vi "HC.vi"() -> ()   [LabVIEW 2022 SP3]
uses:
  <vilib>/numeric/Random Number (Range) I64.vi
  <vilib>/numeric/sub_Random U32.vi
panel:
  in  "TOSS":bool
  in  "Exit":bool
  in  "BOWL":bool
  in  "BAT":bool
  out "RESULT":string
  out "RUNS TO WIN":dbl
  in  "6":bool
  in  "5":bool
  in  "4":bool
  in  "3":bool
  in  "2":bool
  in  "1":bool
  out "BOT RUNS":dbl
  out "PLAYER RUNS":dbl
  out "BOWLING":dbl
  out "BATTING":dbl
  # "SCOREBOARD"
  # "SCOREBOARD"
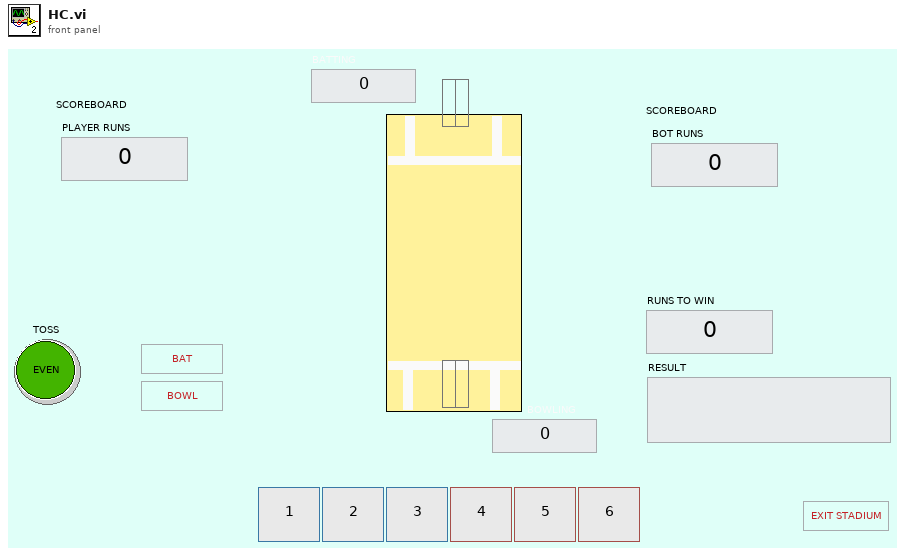
[diagram p1: front panel]
types:
  T1 = cluster{"BAT":bool, "Bowl":bool, "BATTING":dbl, "bowling":dbl, "Target":dbl, "Player Runs":dbl, "Bot Runs":dbl, "Bat CtlRef":refnum<vi>, "Choice":bool[], "RESULT":string, "Choices":dbl, "Innings switched":bool, "Random run":dbl}
  T2 = enum16{"Init", "Poll", "Bat counter", "check wicket", "result", "quit"}
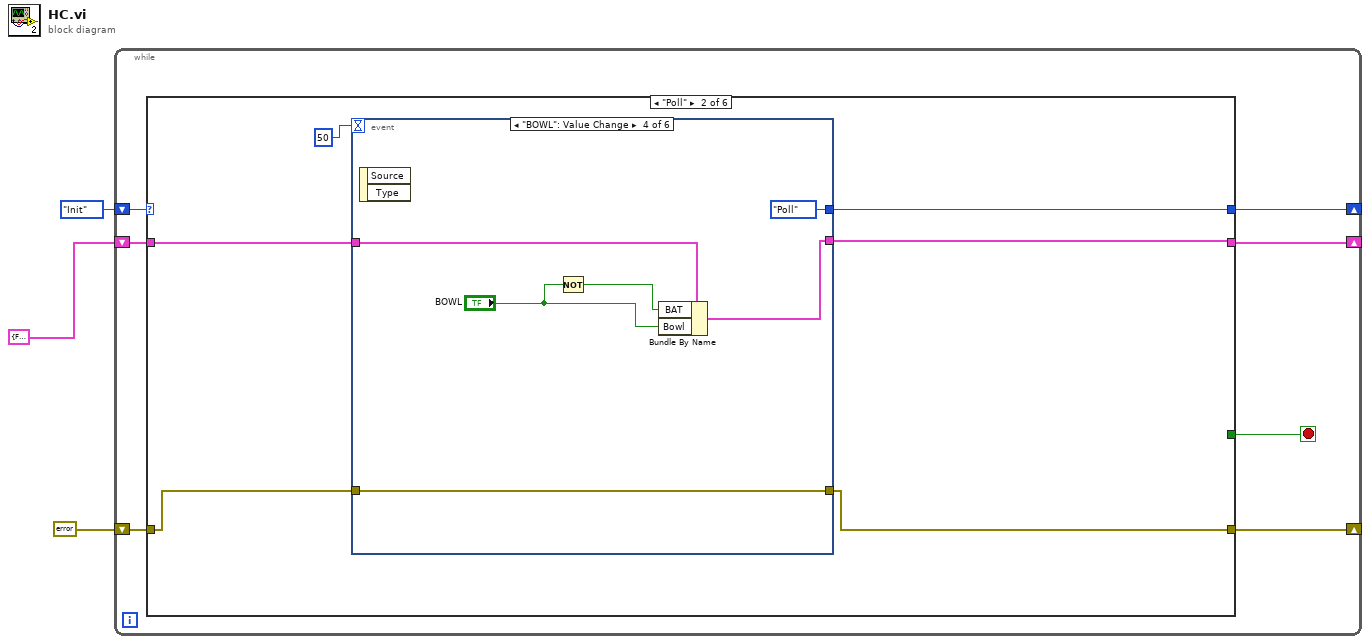
[diagram p0: block diagram]
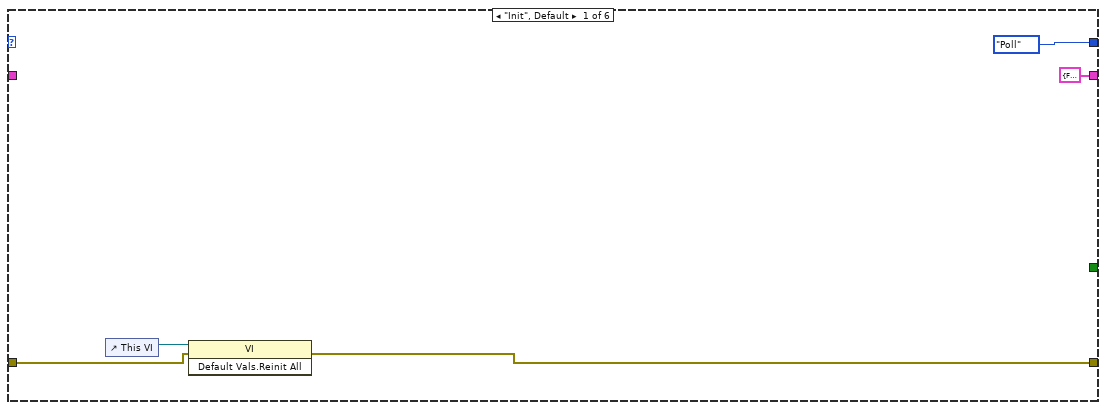
[diagram p2: hidden frame]
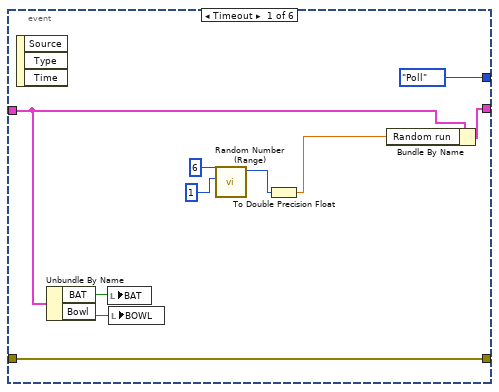
[diagram p3: hidden frame]
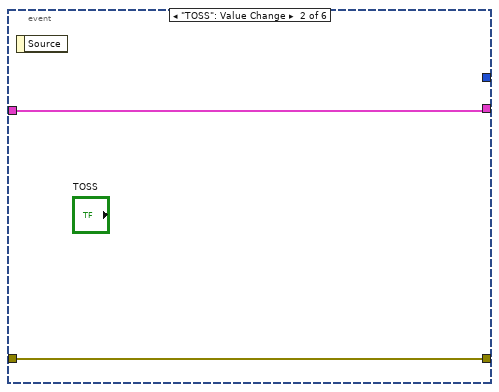
[diagram p4: hidden frame]
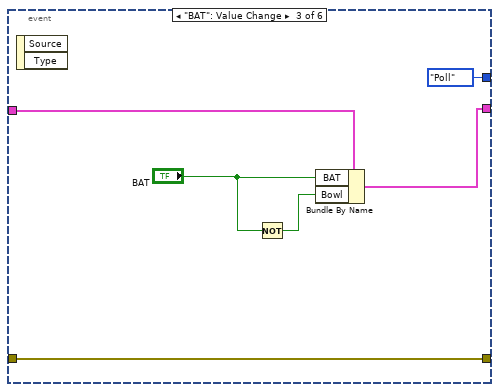
[diagram p5: hidden frame]
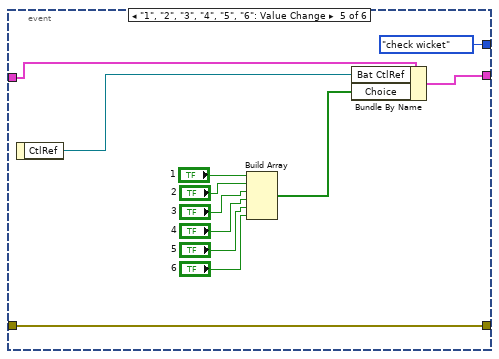
[diagram p6: hidden frame]
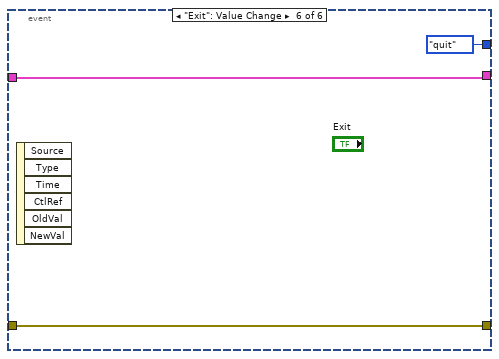
[diagram p7: hidden frame]
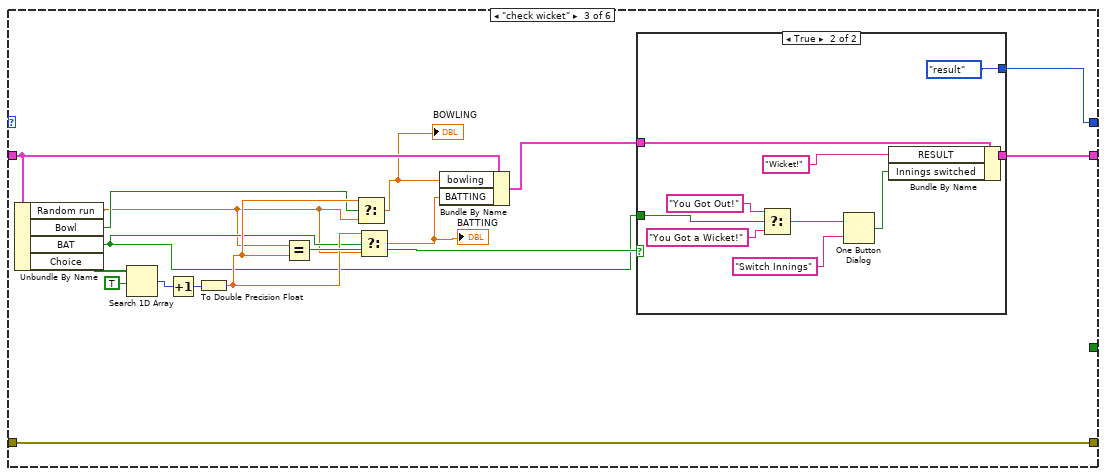
[diagram p8: hidden frame]
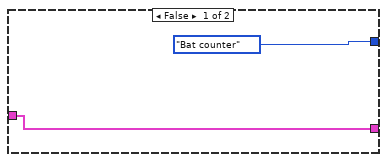
[diagram p9: hidden frame]
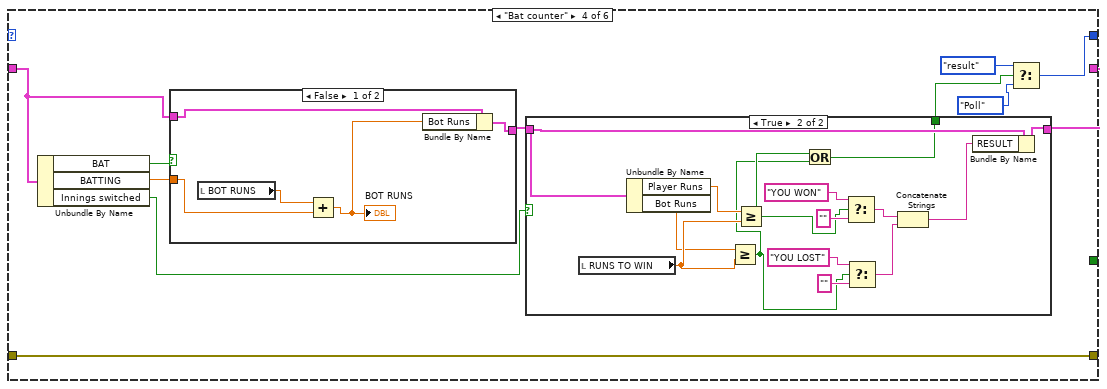
[diagram p10: hidden frame]
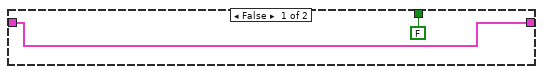
[diagram p11: hidden frame]
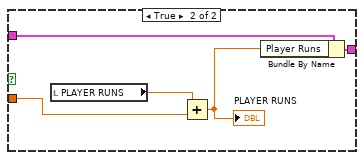
[diagram p12: hidden frame]
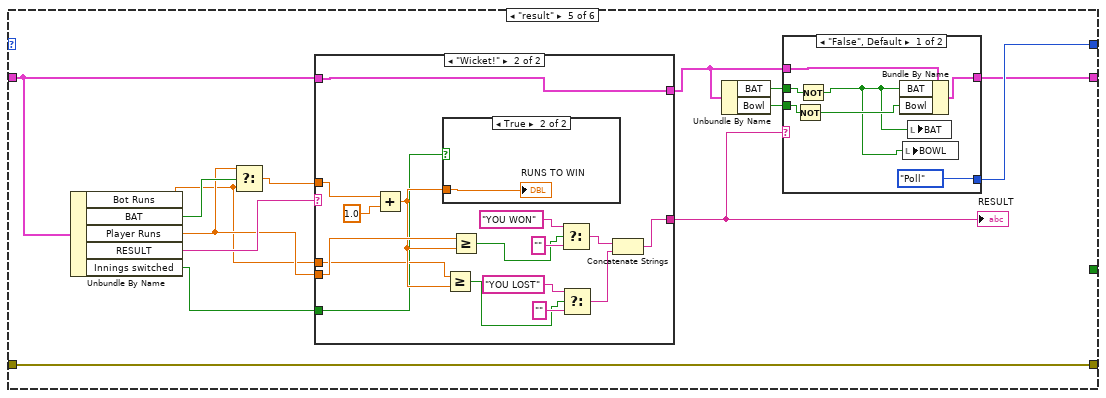
[diagram p13: hidden frame]
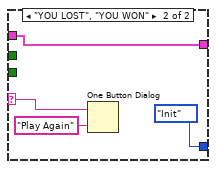
[diagram p14: hidden frame]
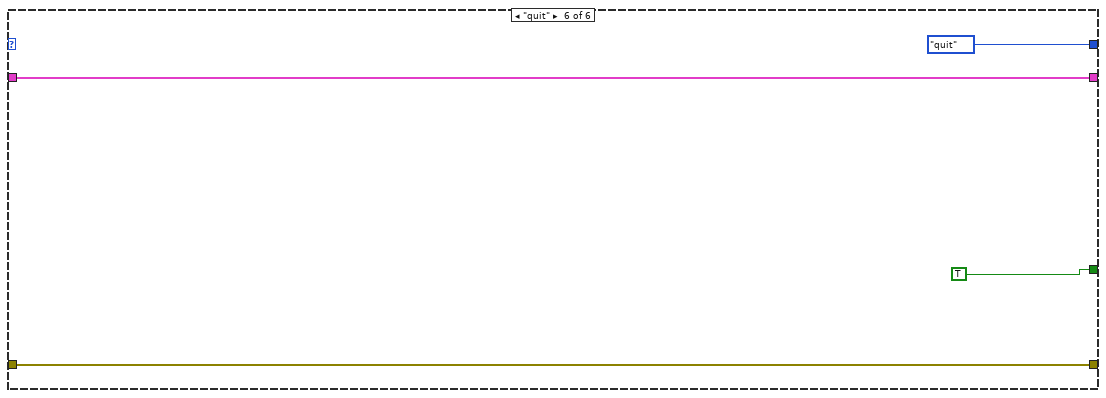
[diagram p17: hidden frame]
diagram:
  n1 = while {
    shift-right: [w9] -> _
    shift-left: T2."Init" -> [w10]
    shift-right: [w8] -> _
    shift-left: T1 {"BAT"=FALSE, "Bowl"=FALSE, "BATTING"=0.0, "bowling"=0.0, "Target"=0.0, "Player Runs"=0.0, "Bot Runs"=0.0, "Bat CtlRef"=refnum, "Choice"=[], "RESULT"="", "Choices"=0.0, "Innings switched"=FALSE, "Random run"=0.0} -> [w7]
    shift-right: [w5] -> _
    shift-left: errorcluster {"status"=FALSE, "code"=0, "source"=""} ("error in (no error)") -> [w6]
    stop <- w4 stop-if-true
    n2 = case shown="\"Poll\"" w10 {
      tunnel: [T2."Poll" ("f") w21 w72 w92 w132 T2."quit" ("f")] -> w9
      tunnel: [T1 {"BAT"=FALSE, "Bowl"=FALSE, "BATTING"=0.0, "bowling"=0.0, "Target"=0.0, "Player Runs"=0.0, "Bot Runs"=0.0, "Bat CtlRef"=refnum, "Choice"=[], "RESULT"="", "Choices"=0.0, "Innings switched"=FALSE, "Random run"=0.0} w19 w63 w94 w130 w174] -> w8
      tunnel: w7 -> [_ w20 w71 w96 w131 w174]
      tunnel: w6 -> [w14 w16 w76 w99 w140 w173]
      tunnel: [w13 w18 w76 w99 w140 w173] -> w5
      tunnel: [_ _ _ _ _ TRUE] -> w4
      frame "Init", Default {
        n3 = control-ref of="This VI"() -> (w15:refnum<vi>)
        n4 = invoke class="VI" method="Default Vals.Reinit All"(reference=w15, error in=w14) -> (error out=w13:errorcluster)  [unwired: 1 in, 2 out]
      }
      frame "Poll" {
        n5 = event shown="[3] \"BOWL\": Value Change" {
          selector: _ -> [_ _ _ _ _ _]
          dyn-events: _ -> [_ _ _ _ _ _]
          timeout: 50 -> [_ _ _ _ _ _]
          tunnel: [T2."Poll" _ T2."Poll" T2."Poll" T2."check wicket" T2."quit"] -> w21
          tunnel: [w26 w33 w37 w43 w56 w60] -> w19
          tunnel: w20 -> [w24 w33 w36 w42 w55 w60]
          tunnel: w16 -> [w30 w32 w39 w45 w53 w59]
          tunnel: [w30 w32 w39 w45 w53 w59] -> w18
          event Timeout {
            n6 = event-data() -> ()  [unwired: 1 in, 3 out]
            n7 = Unbundle By Name(w24) -> ("BAT"=w23:bool, "Bowl"=w22:bool)
            n8 = local write "BAT"(w23) -> ()
            n9 = local write "BOWL"(w22) -> ()
            n10 = call-poly <vilib>:"Random Number (Range).vi"("lower bound (-100)"=i64 1, "upper bound (100)"=i64 6) -> ("number"=w27:i64)  [unwired: 9 in]
            n11 = To Double Precision Float(number=w27) -> (double precision float=w25:dbl)
            n12 = Bundle By Name(cluster=w24, "Random run"=w25) -> (w26:T1)
          }
          event "TOSS": Value Change {
            n13 = event-data() -> ()  [unwired: 1 in, 1 out]
          }
          event "BAT": Value Change {
            n14 = event-data() -> ()  [unwired: 1 in, 2 out]
            n15 = Not(x="BAT") -> (.not. x?=w34:bool)
            n16 = Bundle By Name(cluster=w36, "BAT"="BAT", "Bowl"=w34) -> (w37:T1)
          }
          event "BOWL": Value Change {
            n17 = event-data() -> ()  [unwired: 1 in, 2 out]
            n18 = Not(x="BOWL") -> (.not. x?=w40:bool)
            n19 = Bundle By Name(cluster=w42, "BAT"=w40, "Bowl"="BOWL") -> (w43:T1)
          }
          event "1", "2", "3", "4", "5", "6": Value Change {
            n20 = event-data() -> ("CtlRef"=w54:refnum<vi>)  [unwired: 1 in]
            n21 = Build Array("1", "2", "3", "4", "5", "6") -> (w46:bool[])
            n22 = Bundle By Name(cluster=w55, "Bat CtlRef"=w54, "Choice"=w46) -> (w56:T1)
          }
          event "Exit": Value Change {
            n23 = event-data() -> ()  [unwired: 1 in, 6 out]
          }
        }
      }
      frame "check wicket" {
        n24 = Unbundle By Name(w71) -> ("Random run"=w61:dbl, "Bowl"=w67:bool, "BAT"=w62:bool, "Choice"=w75:bool[])
        n25 = Search 1D Array(1D array=w75, element=TRUE) -> (index of element=w69:i32)  [unwired: 1 in]
        n26 = Increment(x=w69) -> (x+1=w70:i32)
        n27 = To Double Precision Float(number=w70) -> (double precision float=w68:dbl)
        n28 = Equal?(x=w61, y=w68) -> (x = y?=w73:bool)
        n29 = Select(t=w68, s=w67, f=w61) -> (s? t:f=w64:dbl)
        "BOWLING" <- w64
        n30 = Select(t=w68, s=w62, f=w61) -> (s? t:f=w65:dbl)
        "BATTING" <- w65
        n31 = Bundle By Name(cluster=w71, "bowling"=w64, "BATTING"=w65) -> (w66:T1)
        n32 = case shown="True" w73 {
          tunnel: [T2."Bat counter" T2."result" ("f")] -> w72
          tunnel: [w77 w87] -> w63
          tunnel: w66 -> [w77 w86]
          tunnel: w62 -> [_ w84]
          frame False {
          }
          frame True {
            n33 = Select(t="You Got Out!" ("message"), s=w84, f="You Got a Wicket!" ("message")) -> (s? t:f=w81:string)
            n34 = One Button Dialog(message=w81, button name ("OK")="Switch Innings") -> (true=w79:bool)
            n35 = Bundle By Name(cluster=w86, "RESULT"="Wicket!", "Innings switched"=w79) -> (w87:T1)
          }
        }
      }
      frame "Bat counter" {
        n36 = Unbundle By Name(w96) -> ("BAT"=w98:bool, "BATTING"=w97:dbl, "Innings switched"=w89:bool)
        n37 = case shown="False" w98 {
          tunnel: w97 -> [w121 w125]
          tunnel: w96 -> [w119 w124]
          tunnel: [w117 w122] -> w95
          frame False {
            n38 = local read "BOT RUNS"() -> (w120:dbl)
            n39 = Add(x=w120, y=w121) -> (x+y=w118:dbl)
            "BOT RUNS" <- w118
            n40 = Bundle By Name(cluster=w119, "Bot Runs"=w118) -> (w117:T1)
          }
          frame True {
            n41 = local read "PLAYER RUNS"() -> (w126:dbl)
            n42 = Add(x=w126, y=w125) -> (x+y=w123:dbl)
            "PLAYER RUNS" <- w123
            n43 = Bundle By Name(cluster=w124, "Player Runs"=w123) -> (w122:T1)
          }
        }
        n44 = case shown="True" w89 {
          tunnel: w95 -> [w100 w109]
          tunnel: [w100 w106] -> w94
          tunnel: [FALSE w102] -> w90
          frame False {
          }
          frame True {
            n45 = local read "RUNS TO WIN"() -> (w110:dbl)
            n46 = Unbundle By Name(w109) -> ("Player Runs"=w108:dbl, "Bot Runs"=w107:dbl)
            n47 = Greater Or Equal?(x=w107, y=w110) -> (x >= y?=w103:bool)
            n48 = Greater Or Equal?(x=w108, y=w110) -> (x >= y?=w104:bool)
            n49 = Or(x=w104, y=w103) -> (x .or. y?=w102:bool)
            n50 = Select(t="YOU WON" ("RESULT"), s=w104, f="") -> (s? t:f=w112:string)
            n51 = Select(t="YOU LOST" ("RESULT"), s=w103, f="") -> (s? t:f=w111:string)
            n52 = Concatenate Strings(w112, w111) -> (w105:string)
            n53 = Bundle By Name(cluster=w109, "RESULT"=w105) -> (w106:T1)
          }
        }
        n54 = Select(t=T2."result", s=w90, f=T2."Poll") -> (s? t:f=w92:T2)
      }
      frame "result" {
        n55 = Unbundle By Name(w131) -> ("Bot Runs"=w135:dbl, "BAT"=w138:bool, "Player Runs"=w136:dbl, "RESULT"=w139:string, "Innings switched"=w134:bool)
        n56 = Select(t=w136, s=w138, f=w135) -> (s? t:f=w137:dbl)
        n57 = case shown="\"Wicket!\"" w139 {
          selector: w139 -> [w153 _]
          tunnel: w137 -> [_ w169]
          tunnel: w136 -> [_ w167]
          tunnel: [w153 w156] -> w133
          tunnel: w135 -> [_ w163]
          tunnel: w134 -> [_ w155]
          tunnel: w131 -> [w152 w154]
          tunnel: [w152 w154] -> w129
          frame "False", Default {
          }
          frame "Wicket!" {
            n58 = Add(x=w169, y=1.0) -> (x+y=w164:dbl)
            n59 = case shown="True" w155 {
              tunnel: w164 -> [_ w170]
              frame False {
              }
              frame True {
                "RUNS TO WIN" <- w170
              }
            }
            n60 = Greater Or Equal?(x=w163, y=w164) -> (x >= y?=w159:bool)
            n61 = Greater Or Equal?(x=w167, y=w164) -> (x >= y?=w162:bool)
            n62 = Select(t="YOU WON" ("RESULT"), s=w162, f="") -> (s? t:f=w158:string)
            n63 = Select(t="YOU LOST" ("RESULT"), s=w159, f="") -> (s? t:f=w157:string)
            n64 = Concatenate Strings(w158, w157) -> (w156:string)
          }
        }
        "RESULT" <- w133
        n65 = Unbundle By Name(w129) -> ("BAT"=w128:bool, "Bowl"=w127:bool)
        n66 = case shown="\"False\", Default" w133 {
          selector: w133 -> [_ w150]
          tunnel: [T2."Poll" ("f") T2."Init" ("f")] -> w132
          tunnel: w129 -> [w146 w148]
          tunnel: [w145 w148] -> w130
          tunnel: w128 -> [w144 _]
          tunnel: w127 -> [w143 _]
          frame "False", Default {
            n67 = Not(x=w143) -> (.not. x?=w142:bool)
            n68 = Not(x=w144) -> (.not. x?=w141:bool)
            n69 = Bundle By Name(cluster=w146, "BAT"=w141, "Bowl"=w142) -> (w145:T1)
            n70 = local write "BOWL"(w141) -> ()
            n71 = local write "BAT"(w141) -> ()
          }
          frame "YOU LOST", "YOU WON" {
            n72 = One Button Dialog(message=w150, button name ("OK")="Play Again") -> ()  [unwired: 1 out]
          }
        }
      }
      frame "quit" {
      }
    }
  }
